vi "参数设置页.vi"() -> ()   [LabVIEW 2016, in "斯坦道CODMn新电路板.lvlib"]
uses:
  <vilib>/Plasmionique/MB Master/MB_Master/MB_Master.lvclass
  <vilib>/ptbypt/NI_PtbyPt.lvlib
panel:
  in  "标样核查自动补测":bool caption="通讯连接"
  in  "跨度核查自动补测":bool caption="通讯连接"
  in  "零点核查自动补测":bool caption="通讯连接"
  in  "标样核查标液偏差":dbl caption="标样核查标液偏差："
  in  "跨度核查标液偏差":dbl caption="跨度核查标液偏差："
  in  "零点核查标液偏差":dbl caption="零点核查标液偏差："
  out "曲线截距 2":dbl caption="曲线截距：" format="%#.6f"
  out "曲线斜率 2":dbl caption="曲线斜率：" format="%#.6f"
  out "二次多项式系数 2":dbl caption="二次多项式系数：" format="%#.6f"
  out "error out":errorcluster
  in  "公式切换阈值滴定数(0~9999)":dbl
  in  "自动测试量程配置":T2={"水样测试量程模式"=enum."H", "标样核查量程模式"=enum."H", "零点核查量程模式"=enum."H", "跨度核查量程模式"=enum."H", "空白测试量程模式"=enum."H", "平行样测试量程模式"=enum."H", "加标回收量程模式"=enum."H", "空白校准量程模式"=enum."H", "标样校准量程模式"=enum."H"}
  out "数据刷新时间":string
  in  "通讯连接":bool
  out "MB table":enum32{"Serial", "TCP"}(tab)
  in  "请选择串口:":refnum<visa-resource-name>
  in  "IP":string="127.0.0.1"
  in  "PORT":string="1001"
  in  "通信方式选择":enum16{"串口", "TCP"}(ring)
  in  "刷新":bool
  in  "测量模式":T3(ring)
  in  "参数下拉列表":u16(ring) items=["CODMn"]
  in  "量程下拉列表":enum16{"低量程", "高量程"}(ring)
  in  "流程路径":path=path "data/流程.xml"
  out "阈值（高->低）":dbl caption="阈值（高->低）："
  out "阈值（低->高）":dbl caption="阈值（低->高）："
  out "量程下限":dbl caption="量程下限："
  out "量程上限":dbl caption="量程上限："
  out "检出限":dbl caption="检出限："
  out "曲线截距":dbl caption="曲线截距：" format="%#.6f"
  out "曲线斜率":dbl caption="曲线斜率：" format="%#.6f"
  out "二次多项式系数":dbl caption="二次多项式系数：" format="%#.6f"
  out "消解时长":dbl caption="消解时长："
  out "消解温度":dbl caption="消解温度："
  out "测量精度":dbl caption="测量精度："
  in  "标样核查标液浓度":dbl caption="标样核查标液浓度："
  in  "跨度核查标液浓度":dbl caption="跨度核查标液浓度："
  in  "零点核查标液浓度":dbl caption="零点核查标液浓度："
  in  "跨度值":dbl caption="跨度值："
  # "日质控自动补测设置"
  # "±"
  # "%"
  # "%"
  # "第一段线性公式"
  # "第二段线性公式"
  # "mg/L"
  # "mg/L"
  # "mg/L"
  # "mg/L"
  # "mg/L"
  # "min"
  # "℃"
  # "mg/L"
  # "mg/L"
  # "mg/L"
  # "mg/L"
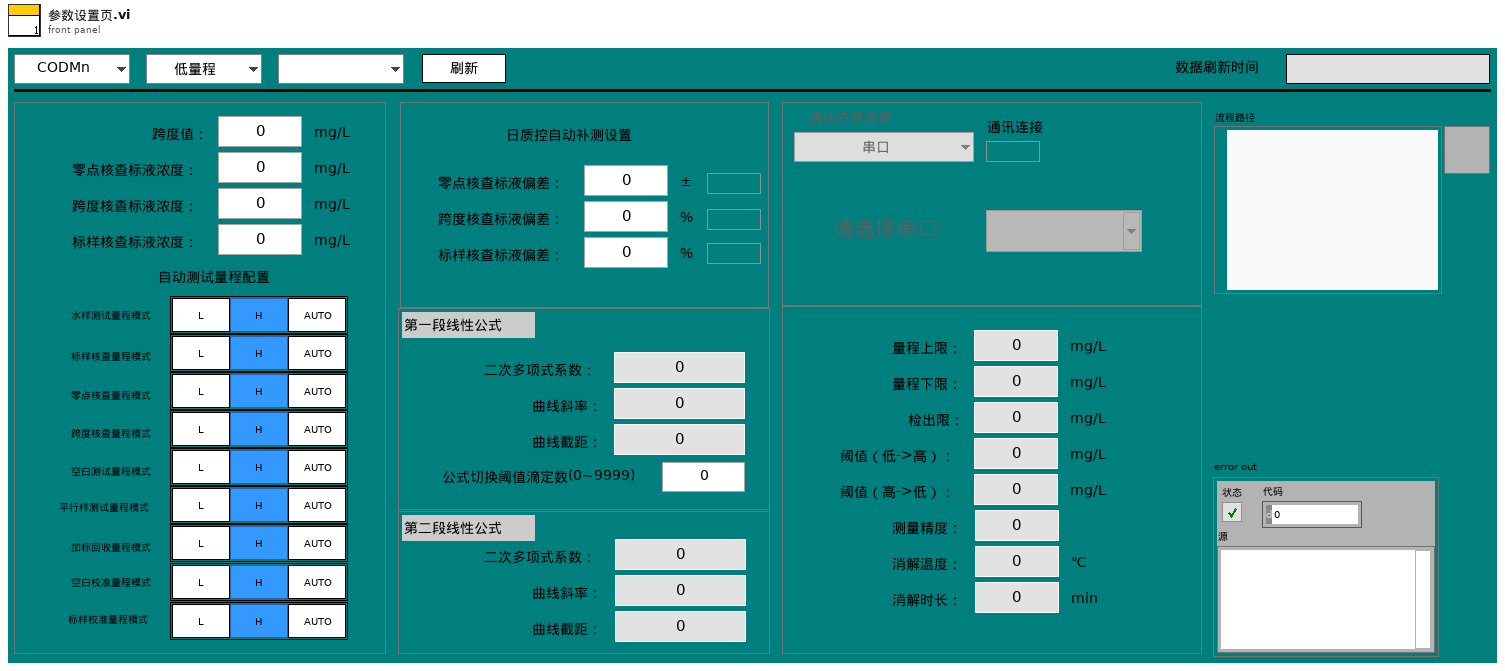
[diagram p1: front panel]
types:
  T1 = typedef "量程选择控件.ctl" = enum32{"L", "H", "AUTO"}
  T2 = cluster{"水样测试量程模式":T1, "标样核查量程模式":T1, "零点核查量程模式":T1, "跨度核查量程模式":T1, "空白测试量程模式":T1, "平行样测试量程模式":T1, "加标回收量程模式":T1, "空白校准量程模式":T1, "标样校准量程模式":T1}
  T3 = enum16{"", "水样测量", "标样核查", "零点核查", "跨度核查", "空白测试", "平行样测试", "加标回收"}
  T4 = enum8{"Enabled", "Disabled", "Disabled and Grayed Out"}
  T5 = cluster{"系统时间":timestamp, "工作状态":u16, "测量模式":enum16{"待机", "连续模式", "周期模式", "定点模式", "受控模式", "手动模式"}, "告警代码":u16, "故障代码":u16, "日志代码":u16, "软件版本":u16, "A":sgl, "B":sgl, "K":sgl, "当前滴定数":sgl, "T":sgl, "H":sgl, "id":u16, "flowid":u16, "量程":u16, "加热实时温度":sgl, "当前ORP值":sgl, "运行时间":sgl, "当前步骤剩余时间":sgl, "结束滴定数":sgl, "注射泵保温温度":sgl, "匹配滴定数X0":u16, "X^2":sgl, "X":sgl, "B 2":sgl, "光值1":sgl, "光值2":sgl, "光值3":sgl, "光值4":sgl, "光值5":sgl, "光值6":sgl, "光值7":sgl, "光值8":sgl}
  T6 = cluster{"检出限":dbl, "测量精度":dbl, "上限":dbl, "下限":dbl, "阈值（低->高）":dbl, "阈值（高->低）":dbl}
  T7 = cluster{"标液浓度1":dbl, "测量吸光度1":dbl, "样品1启用":bool, "标液浓度2":dbl, "测量吸光度2":dbl, "样品2启用":bool, "标液浓度3":dbl, "测量吸光度3":dbl, "样品3启用":bool, "标液浓度4":dbl, "测量吸光度4":dbl, "样品4启用":bool, "标液浓度5":dbl, "测量吸光度5":dbl, "样品5启用":bool, "模型":enum32{"线性", "多项式", "折线"}, "精度":dbl, "XY图":cluster{"X Values":dbl[], "Y Values":dbl[]}[], "拟合公式":string, "r^2":dbl, "标样一校准时间":timestamp, "标样二校准时间":timestamp, "标样三校准时间":timestamp, "标样四校准时间":timestamp, "标样五校准时间":timestamp, "二次方程":cluster{"c":dbl, "x":dbl, "x^2":dbl}, "标定时间":timestamp, "拟合公式 2":string, "r^2 2":dbl}[][]
  T8 = cluster{"运行模式":enum16{"维护模式", "常规模式", "应急模式", "质控模式"}, "质控频次":enum16{"关闭", "每天", "星期一", "星期二", "星期三", "星期四", "星期五", "星期六", "星期日"}, "空白核查时间":u16, "跨度核查时间":u16, "测量间隔":u16}
  T9 = cluster{"标液浓度1":dbl, "测量吸光度1":dbl, "样品1启用":bool, "标液浓度2":dbl, "测量吸光度2":dbl, "样品2启用":bool, "标液浓度3":dbl, "测量吸光度3":dbl, "样品3启用":bool, "标液浓度4":dbl, "测量吸光度4":dbl, "样品4启用":bool, "标液浓度5":dbl, "测量吸光度5":dbl, "样品5启用":bool, "模型":enum32{"线性", "多项式", "折线"}, "精度":dbl, "XY图":cluster{"X Values":dbl[], "Y Values":dbl[]}[], "拟合公式":string, "r^2":dbl, "标样一校准时间":timestamp, "标样二校准时间":timestamp, "标样三校准时间":timestamp, "标样四校准时间":timestamp, "标样五校准时间":timestamp, "二次方程":cluster{"c":dbl, "x":dbl, "x^2":dbl}, "标定时间":timestamp, "拟合公式 2":string, "r^2 2":dbl}
  T10 = cluster{"测量量程":sgl, "测量检出限":sgl, "测量精度":sgl, "测量间隔":sgl, "消解温度":sgl, "消解时长":sgl, "三项式系数":sgl, "二次多项式系数":sgl, "曲线斜率":sgl, "曲线截距":sgl, "线性相关系数":sgl, "空白校准时间":timestamp, "标样校准时间":timestamp, "测量信号值":sgl, "稀释倍数":sgl, "量程系数":sgl}
  T11 = cluster{"偏心轮校准参数":dbl, "运行速度(修改需要重启)":u16, "加热温度(校准参数) ":dbl, "告警温度":dbl, "加热超时时间:(单位/秒)":dbl, "K p":dbl, "K i":dbl, "K d":dbl, "ILimitUp":dbl, "ILimitDown":dbl}
  T12 = cluster{"泵类型":u8, "阀数量":u8, "纯水通道":u8, "废液通道":u8, "进样速度":u16, "出样速度":u16, "滴定速度":u16, "注射泵保温温度L":u8, "注射泵保温温度H":u8, "注射泵加热超时时间":u16, "是否存在液位检测板":u16, "A值告警下限值":u16, "A值告警上限值":u16, "B值告警下限值":u16, "B值告警上限值":u16, "AB跨度告警值":u16, "阀配置:":u8, "滴定等待时间":u16, "滴定吸光度斜率":dbl}
  T13 = cluster{"跨度值":dbl, "零点标准液浓度":dbl, "跨度标准液浓度":dbl, "标准液标准浓度":dbl, "零点标准液偏差":dbl, "跨度标准液偏差":dbl, "标准液标准偏差":dbl}
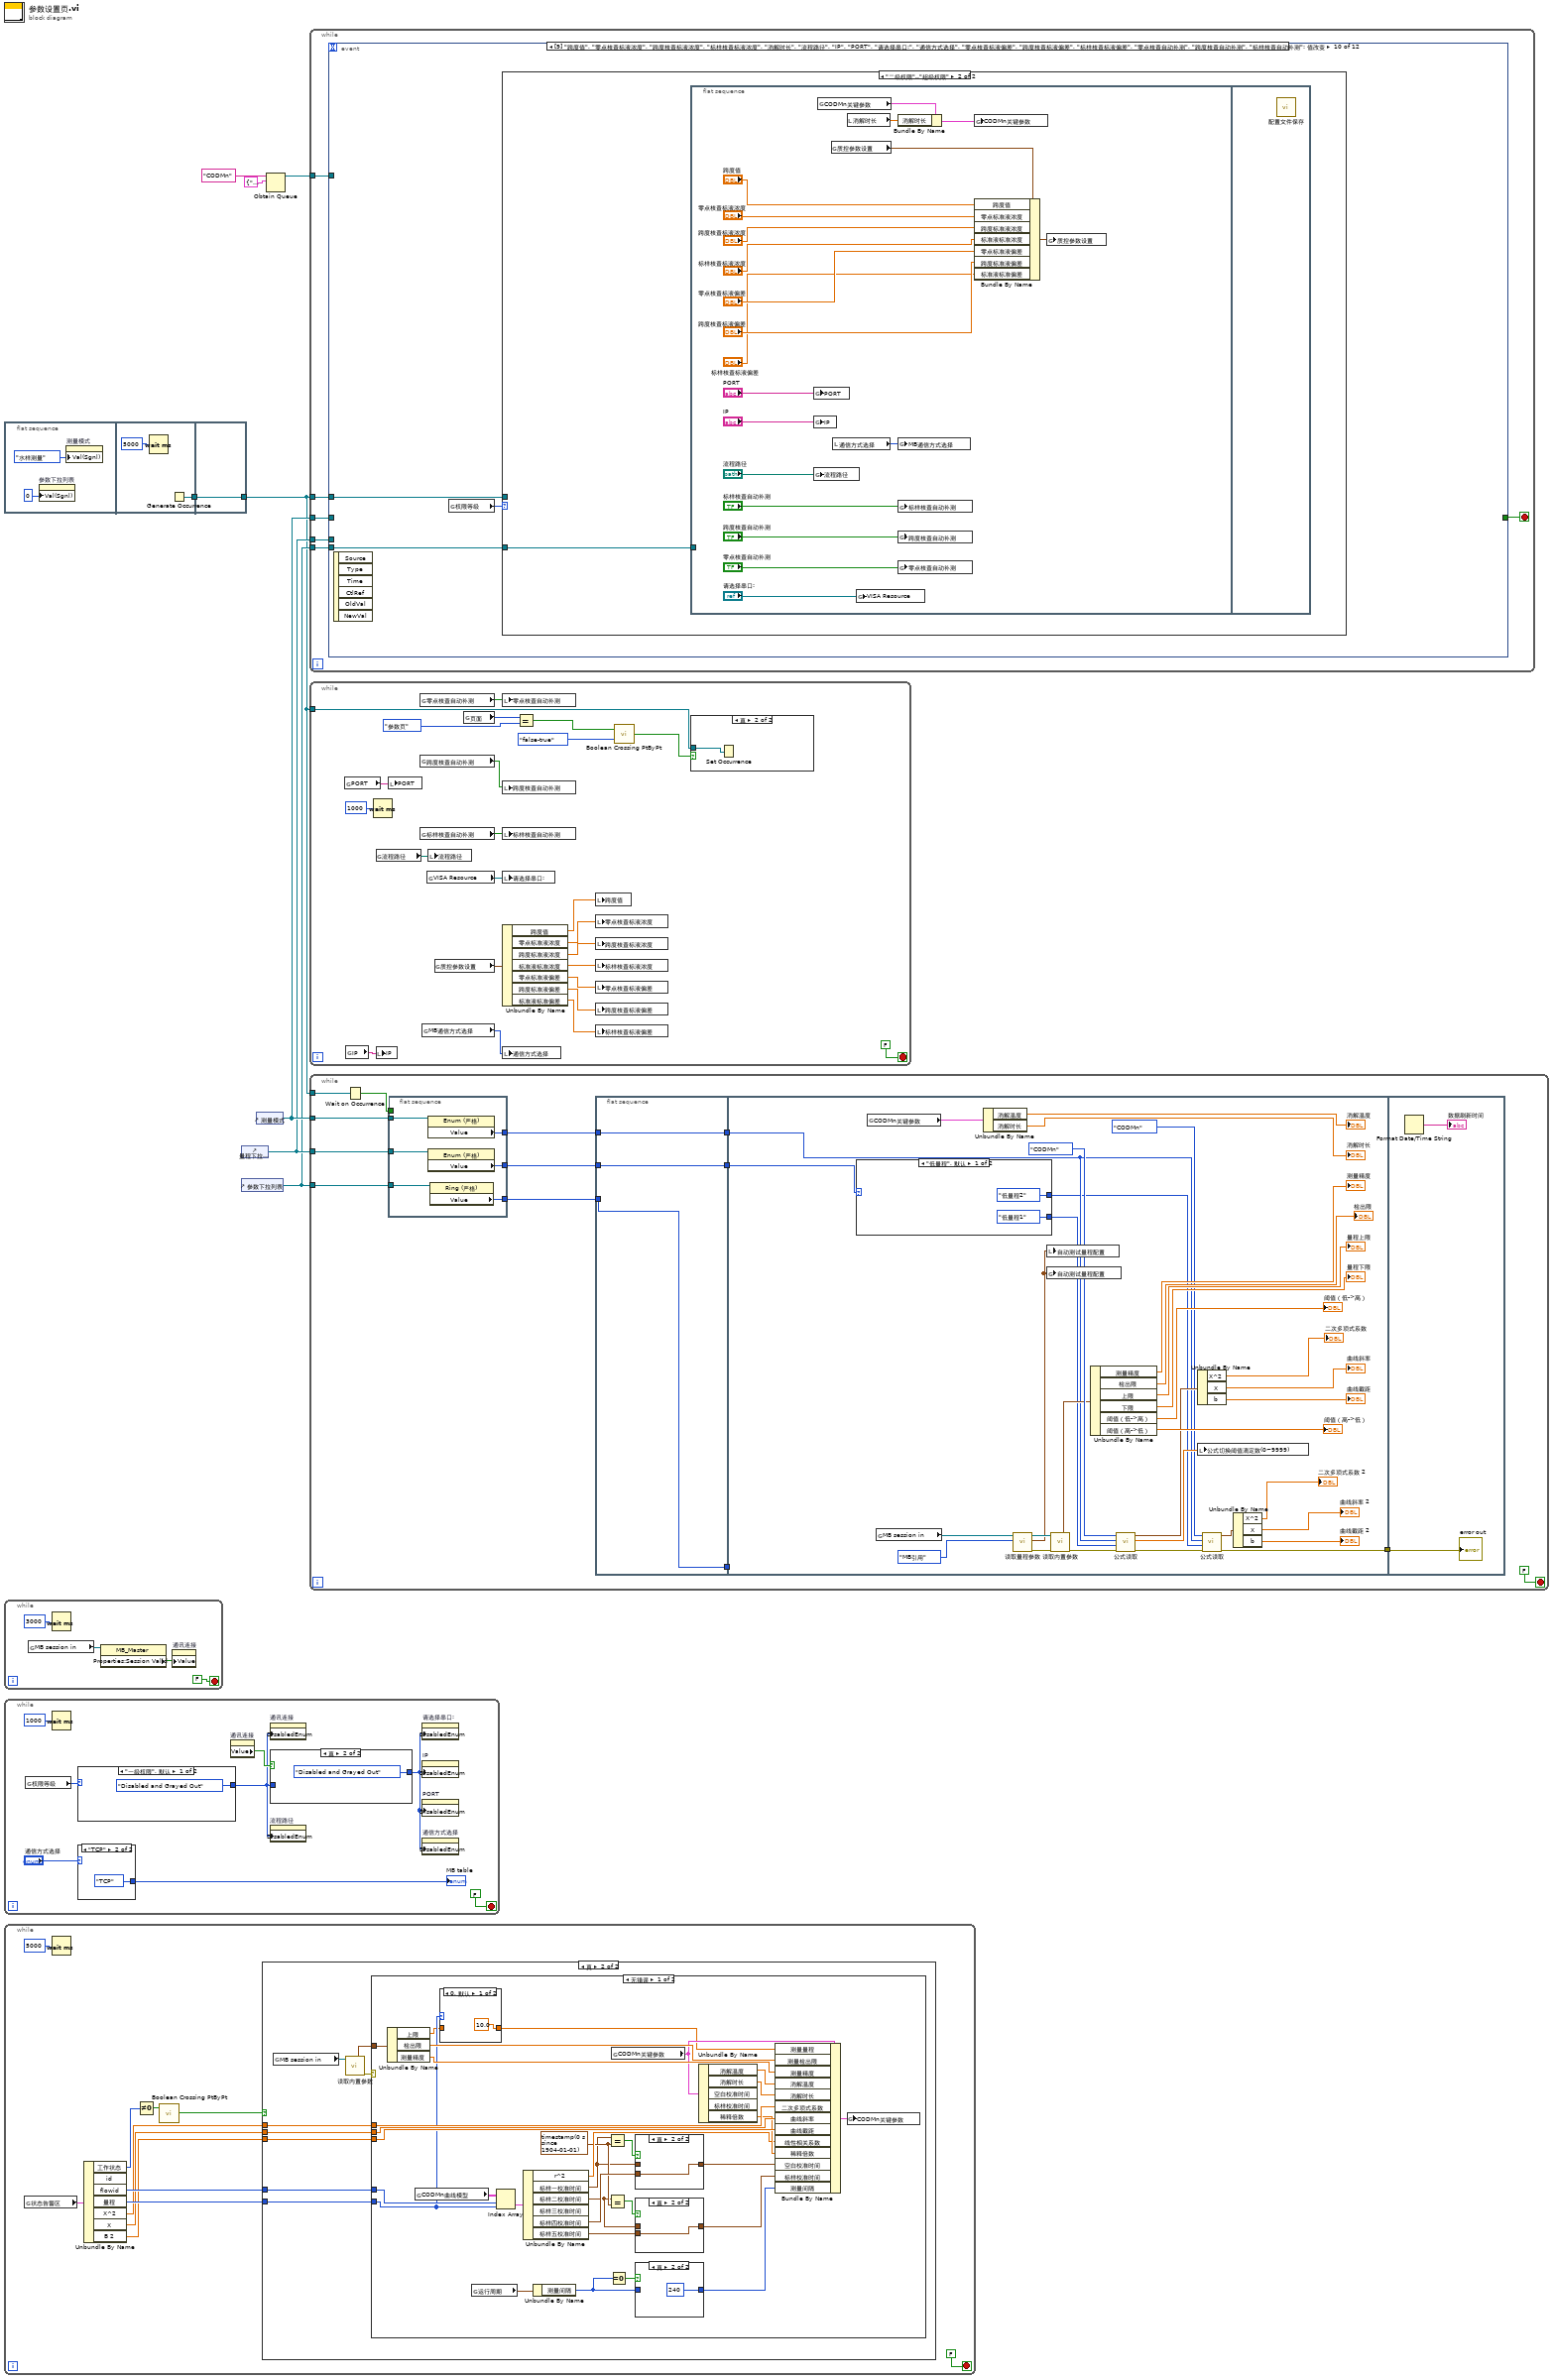
[diagram p0: block diagram]
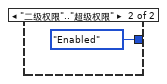
[diagram p9: hidden frame]
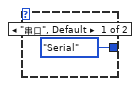
[diagram p10: hidden frame]
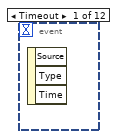
[diagram p12: hidden frame]
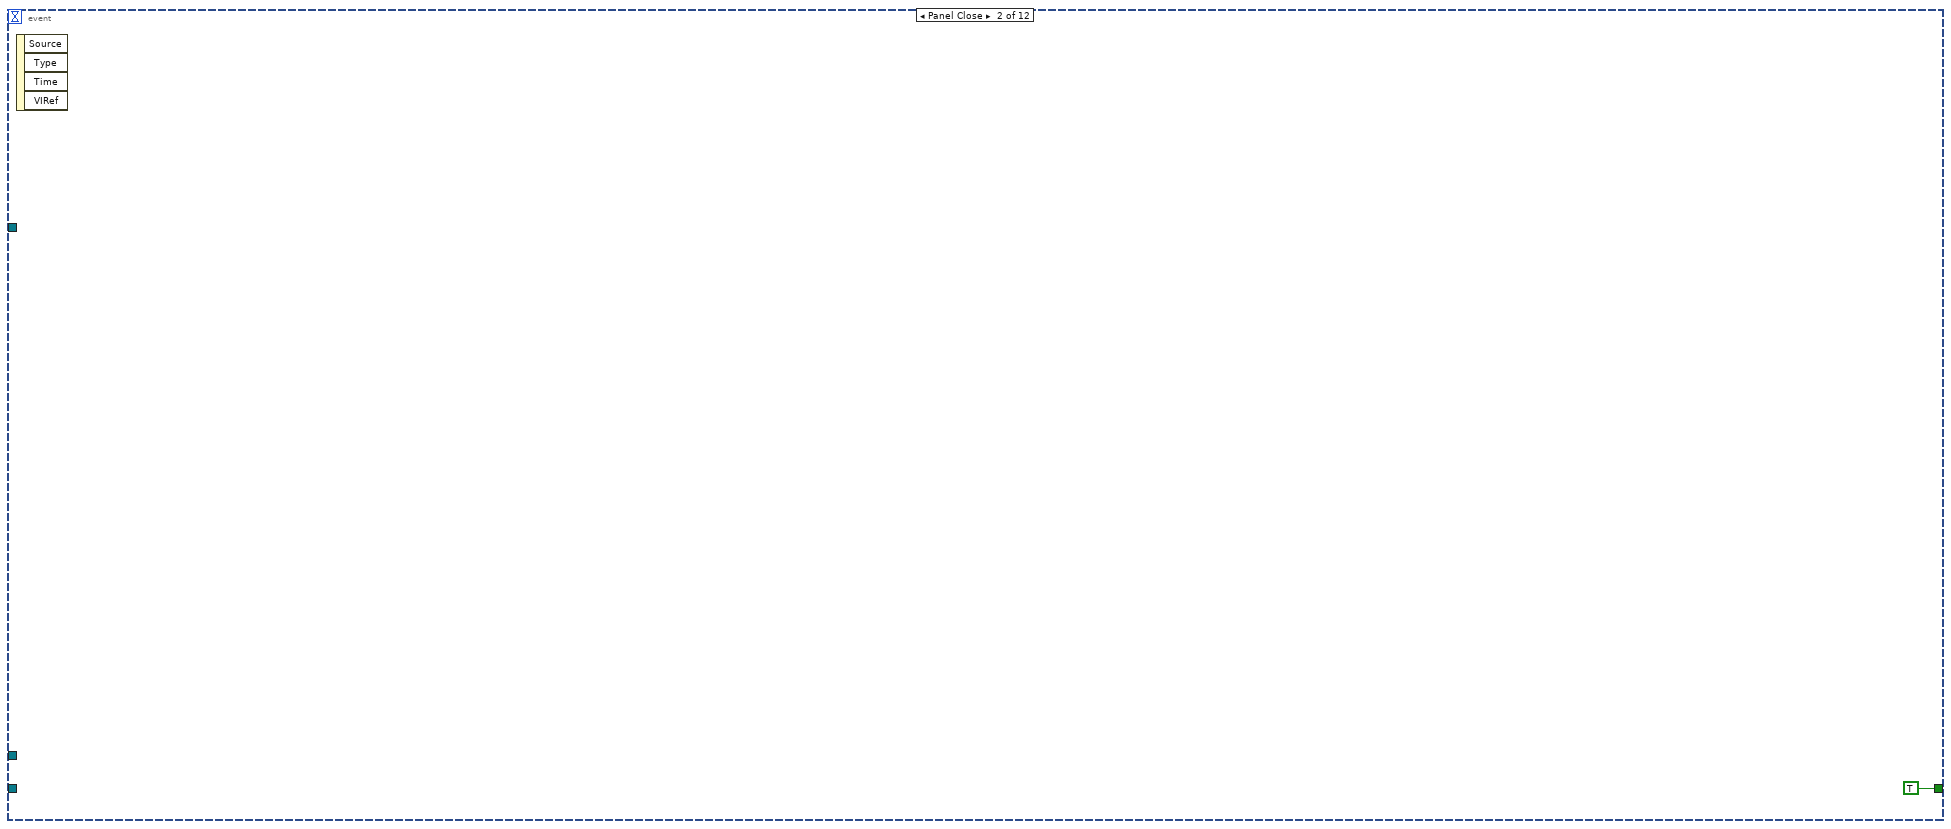
[diagram p13: hidden frame]
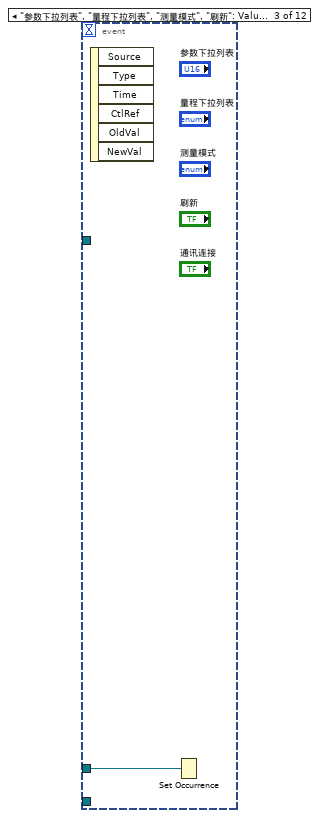
[diagram p14: hidden frame]
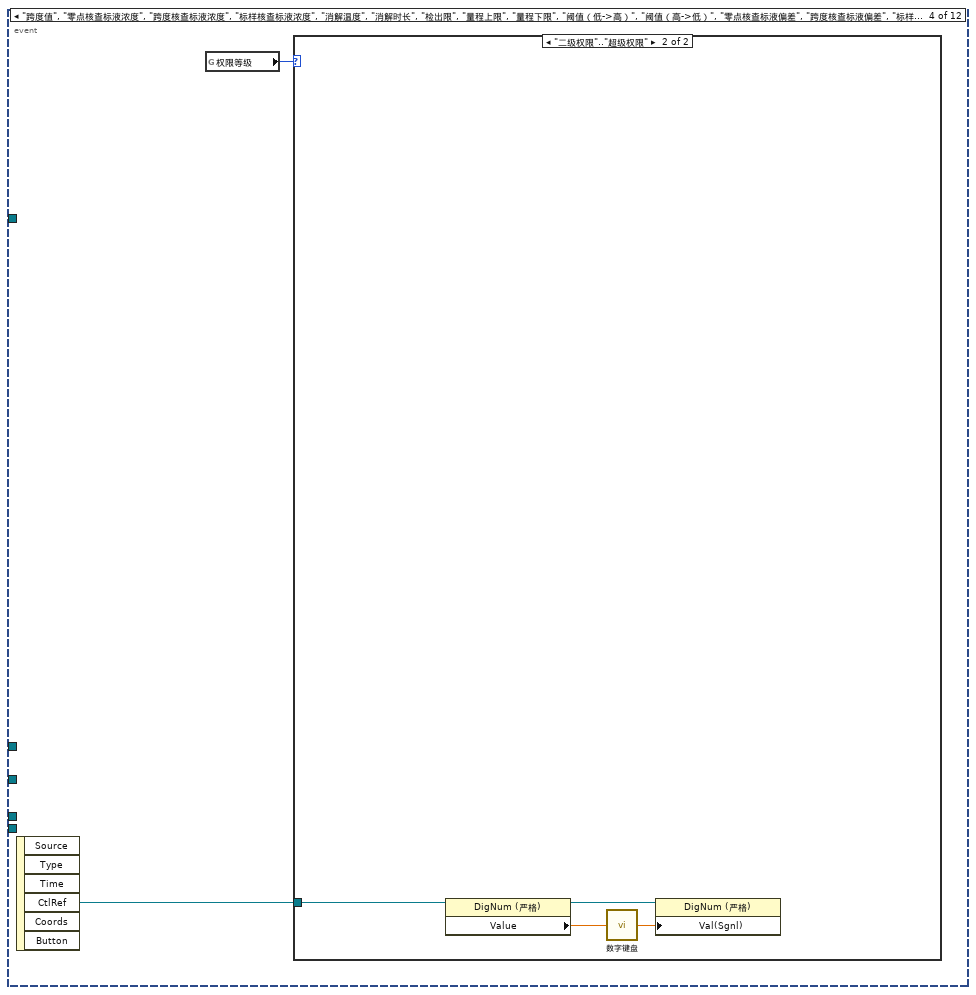
[diagram p15: hidden frame]
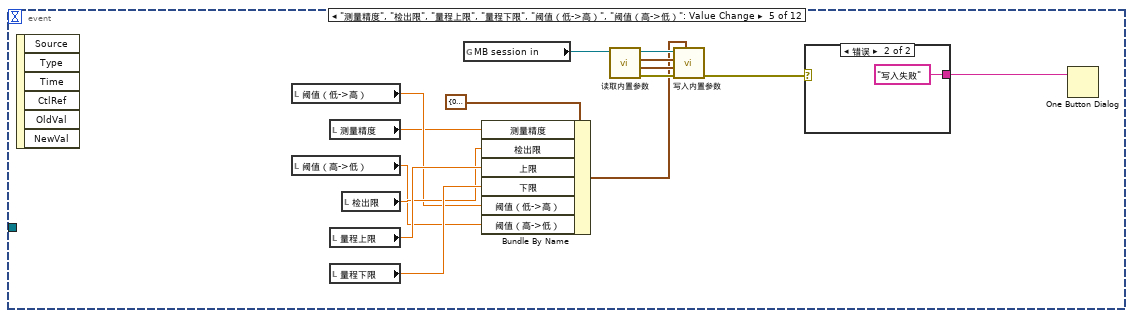
[diagram p17: hidden frame]
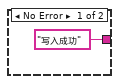
[diagram p18: hidden frame]
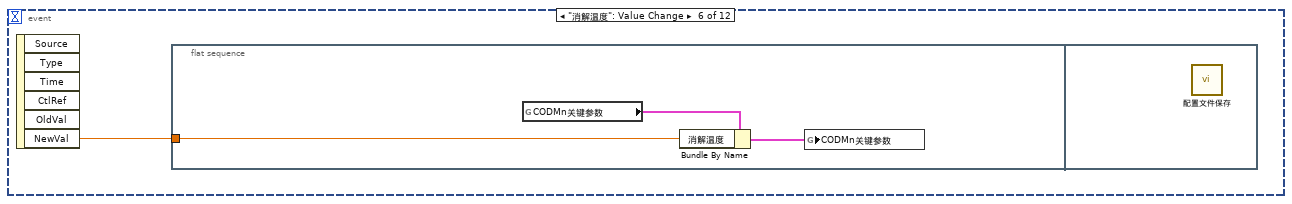
[diagram p19: hidden frame]
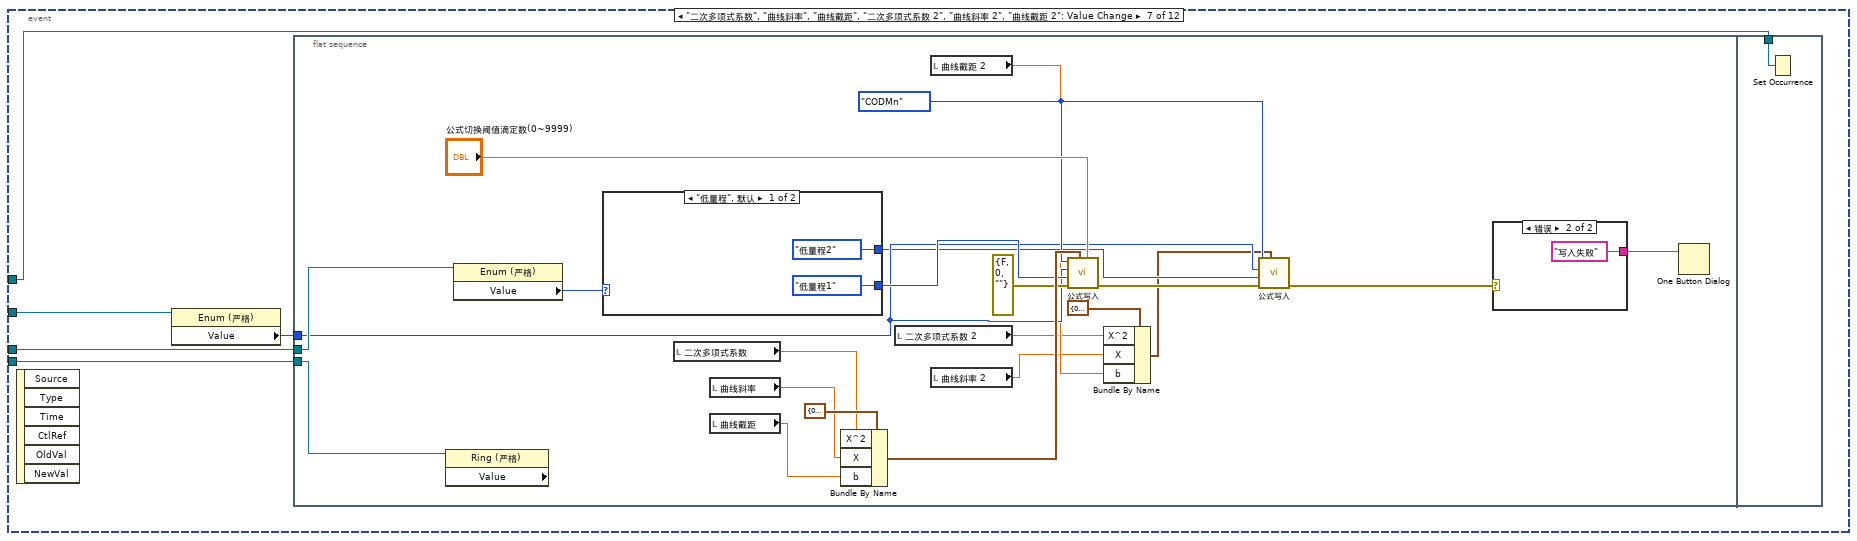
[diagram p20: hidden frame]
diagram:
  n1 = flat-sequence {
    tunnel: [w12] -> w8
    tunnel: [w13] -> w1
    tunnel: w8 -> [w13]
    frame #0 {
      n2 = property on="参数下拉列表" class="Ring (严格)"("Val(Sgnl)"=u16 0 ("值(信号)")) -> ()  [unwired: 2 in, 2 out]
      n3 = property on="测量模式" class="Enum (严格)"("Val(Sgnl)"=T3."水样测量" ("值(信号)")) -> ()  [unwired: 2 in, 2 out]
    }
    frame #1 {
      n4 = Wait (ms)(milliseconds to wait=u32 5000 ("等待时间（毫秒）")) -> ()  [unwired: 1 out]
      n5 = Generate Occurrence() -> (w12:refnum<k4>)
    }
    frame #2 {
    }
  }
  n6 = while {
    stop <- FALSE stop-if-true
    n7 = global read "VARCODMn全局变量.vi" "MB session in"() -> (w16:refnum<class "MB_Master.lvclass">)
    n8 = Wait (ms)(milliseconds to wait=u32 3000 ("等待时间（毫秒）")) -> ()  [unwired: 1 out]
    n9 = property class="MB_Master"(reference=w16) -> ("Properties:Session Valid"=w15:bool)  [unwired: 1 in, 2 out]
    n10 = property on="通讯连接" class="Bool (严格)"("Value"=w15) -> ()  [unwired: 2 in, 2 out]
  }
  n11 = while {
    stop <- FALSE stop-if-true
    n12 = global read "VARCODMn全局变量.vi" "权限等级"() -> (w18:enum16{"一级权限", "二级权限", "三级权限", "超级权限"})
    n13 = Wait (ms)(milliseconds to wait=u32 1000 ("等待时间（毫秒）")) -> ()  [unwired: 1 out]
    n14 = case shown="\"一级权限\", 默认" w18 {
      tunnel: [T4."Disabled and Grayed Out" ("禁用") T4."Enabled" ("禁用")] -> w19
      frame "一级权限", Default {
      }
      frame "二级权限".."超级权限" {
      }
    }
    n15 = case shown="\"TCP\"" "通信方式选择" {
      tunnel: [enum32{"Serial", "TCP"}."Serial" ("MB table") enum32{"Serial", "TCP"}."TCP" ("MB table")] -> w21
      frame "串口", Default {
      }
      frame "TCP" {
      }
    }
    "MB table" <- w21
    n16 = property on="通讯连接" class="Bool (严格)"() -> ("Value"=w23:bool)  [unwired: 2 in, 2 out]
    n17 = property on="通讯连接" class="Bool (严格)"("DisabledEnum"=w19) -> ()  [unwired: 2 in, 2 out]
    n18 = case shown="真" w23 {
      tunnel: [w30 T4."Disabled and Grayed Out" ("禁用")] -> w22
      tunnel: w19 -> [w30 _]
      frame False {
      }
      frame True {
      }
    }
    n19 = property on="流程路径" class="Path"("DisabledEnum"=w19) -> ()  [unwired: 2 in, 2 out]
    n20 = property on="请选择串口:" class="VISAName"("DisabledEnum"=w22) -> ()  [unwired: 2 in, 2 out]
    n21 = property on="IP" class="Str"("DisabledEnum"=w22) -> ()  [unwired: 2 in, 2 out]
    n22 = property on="PORT" class="Str"("DisabledEnum"=w22) -> ()  [unwired: 2 in, 2 out]
    n23 = property on="通信方式选择" class="Enum (严格)"("DisabledEnum"=w22) -> ()  [unwired: 2 in, 2 out]
  }
  n24 = while {
    stop <- FALSE stop-if-true
    n25 = global read "VARCODMn全局变量.vi" "状态告警区"() -> (w42:T5)
    n26 = Wait (ms)(milliseconds to wait=u32 5000 ("等待时间（毫秒）")) -> ()  [unwired: 1 out]
    n27 = Unbundle By Name(w42) -> ("工作状态"=w41:u16, "flowid"=w35:u16, "量程"=w36:u16, "X^2"=w34:sgl, "X"=w33:sgl, "B 2"=w32:sgl)  [unwired: 1 out]
    n28 = Not Equal To 0?(x=w41) -> (x != 0?=w40:bool)
    n29 = call <vilib>:"Boolean Crossing PtByPt.vi"("input"=w40) -> ("crossing"=w39:bool)  [unwired: 2 in]
    n30 = case shown="真" w39 {
      tunnel: w36 -> [_ w48]
      tunnel: w35 -> [_ w47]
      tunnel: w34 -> [_ w46]
      tunnel: w33 -> [_ w45]
      tunnel: w32 -> [_ w44]
      frame False {
      }
      frame True {
        n31 = global read "VARCODMn全局变量.vi" "MB session in"() -> (w50:refnum<class "MB_Master.lvclass">)
        n32 = call "读取内置参数.vi"("MB session in"=w50) -> ("error out"=w43:errorcluster, "量程参数读取"=w49:T6)  [unwired: 6 in, 3 out]
        n33 = case shown="无错误" w43 {
          tunnel: w49 -> [w81 _]
          tunnel: w46 -> [w80 _]
          tunnel: w45 -> [w79 _]
          tunnel: w44 -> [w78 _]
          tunnel: w48 -> [w53 _]
          tunnel: w47 -> [w71 _]
          frame No Error {
            w60 = timestamp(0 s since 1904-01-01) ("y")
            n34 = Unbundle By Name(w81) -> ("上限"=w52:dbl, "检出限"=w77:dbl, "测量精度"=w76:dbl)
            n35 = global read "校准数据全局变量.vi" "CODMn曲线模型"() -> (w72:T7)
            n36 = case shown="0, 默认" w53 {
              tunnel: w52 -> [_ w83]
              tunnel: [10.0 ("上限") w83] -> w51
              frame 0, Default {
              }
              frame 1 {
              }
            }
            n37 = global read "CODMn断电保存全局变量.vi" "运行周期"() -> (w67:T8)
            n38 = Index Array(array=w72, index (row)=w71, index (col)=w53) -> (element=w70:T9)
            n39 = Unbundle By Name(w70) -> ("r^2"=w68:dbl, "标样一校准时间"=w56:timestamp, "标样二校准时间"=w57:timestamp, "标样四校准时间"=w61:timestamp, "标样五校准时间"=w58:timestamp)  [unwired: 1 out]
            n40 = Unbundle By Name(w67) -> ("测量间隔"=w63:u16)
            n41 = Equal?(x=w56, y=w60) -> (x = y?=w62:bool)
            n42 = Equal?(x=w57, y=w60) -> (x = y?=w59:bool)
            n43 = Equal To 0?(x=w63) -> (x = 0?=w65:bool)
            n44 = global read "CODMn断电保存全局变量.vi" "CODMn关键参数"() -> (w66:T10)
            n45 = case shown="真" w62 {
              tunnel: w61 -> [_ w87]
              tunnel: [w86 w87] -> w55
              tunnel: w56 -> [w86 _]
              frame False {
              }
              frame True {
              }
            }
            n46 = case shown="真" w59 {
              tunnel: w58 -> [_ w85]
              tunnel: [w84 w85] -> w54
              tunnel: w57 -> [w84 _]
              frame False {
              }
              frame True {
              }
            }
            n47 = case shown="真" w65 {
              tunnel: [w88 u16 240 ("测量间隔")] -> w64
              tunnel: w63 -> [w88 _]
              frame False {
              }
              frame True {
              }
            }
            n48 = Unbundle By Name(w66) -> ("消解温度"=w75:sgl, "消解时长"=w74:sgl, "稀释倍数"=w69:sgl)  [unwired: 2 out]
            n49 = Bundle By Name(cluster=w66, "测量量程"=w51, "测量检出限"=w77, "测量精度"=w76, "消解温度"=w75, "消解时长"=w74, "二次多项式系数"=w80, "曲线斜率"=w79, "曲线截距"=w78, "线性相关系数"=w68, "稀释倍数"=w69, "空白校准时间"=w55, "标样校准时间"=w54, "测量间隔"=w64) -> (w73:T10)
            n50 = global write "CODMn断电保存全局变量.vi" "CODMn关键参数"(w73) -> ()
          }
          frame Error {
          }
        }
      }
    }
  }
  n51 = control-ref of="量程下拉列表"() -> (w4:refnum<vi>)
  n52 = control-ref of="参数下拉列表"() -> (w3:refnum<vi>)
  n53 = control-ref of="测量模式"() -> (w5:refnum<vi>)
  n54 = Obtain Queue(name (unnamed)="CODMn" ("名称（未命名）"), element data type=cluster{"命令":string, "data":variant} {"命令"="", "data"=variant}) -> (queue out=w6:refnum<queue>)  [unwired: 3 in, 2 out]
  n55 = while {
    tunnel: w1 -> [w94]
    tunnel: w3 -> [w93]
    tunnel: w6 -> [w92]
    tunnel: w5 -> [w91]
    tunnel: w4 -> [w90]
    stop <- w95 stop-if-true
    n56 = event shown="[9] \"跨度值\", \"零点核查标液浓度\", \"跨度核查标液浓度\", \"标样核查标液浓度\", \"消解时长\", \"流程路径\", \"IP\", \"PORT\", \"请选择串口:\", \"通信方式选择\", \"零点核查标液偏差\", \"跨度核查标液偏差\", \"标样核查标液偏差\", \"零点核查自动补测\", \"跨度核查自动补测\", \"标样核查自动补测\": 值改变" {
      selector: _ -> [_ _ _ _ _ _ _ _ _ _ _ _]
      dyn-events: _ -> [_ _ _ _ _ _ _ _ _ _ _ _]
      timeout: _ -> [_ _ _ _ _ _ _ _ _ _ _ _]
      tunnel: [_ TRUE _ _ _ _ _ _ _ _ _ _] -> w95
      tunnel: w94 -> [_ _ w97 _ _ _ w125 _ _ w172 w197 _]
      tunnel: w93 -> [_ _ _ _ _ _ w129 _ _ w174 _ _]
      tunnel: w92 -> [_ _ _ _ _ _ _ _ _ _ _ w203]
      tunnel: w91 -> [_ _ _ _ _ _ w128 _ _ _ _ _]
      tunnel: w90 -> [_ _ _ _ _ _ w126 _ _ _ _ _]
      event Timeout {
        n57 = event-data() -> ()  [unwired: 1 in, 3 out]
      }
      event Panel Close {
        n58 = event-data() -> ()  [unwired: 1 in, 4 out]
      }
      event "参数下拉列表", "量程下拉列表", "测量模式", "刷新": Value Change {
        n59 = event-data() -> ()  [unwired: 1 in, 6 out]
        n60 = Set Occurrence(w97) -> ()
      }
      event "跨度值", "零点核查标液浓度", "跨度核查标液浓度", "标样核查标液浓度", "消解温度", "消解时长", "检出限", "量程上限", "量程下限", "阈值（低->高）", "阈值（高->低）", "零点核查标液偏差", "跨度核查标液偏差", "标样核查标液偏差": Mouse Down {
        n61 = event-data() -> ("CtlRef"=w99:refnum<vi>)  [unwired: 1 in, 5 out]
        n62 = global read "VARCODMn全局变量.vi" "权限等级"() -> (w98:enum16{"一级权限", "二级权限", "三级权限", "超级权限"})
        n63 = case shown="\"二级权限\"..\"超级权限\"" w98 {
          tunnel: w99 -> [_ w103]
          frame "一级权限", Default {
          }
          frame "二级权限".."超级权限" {
            n64 = property class="DigNum (严格)"(reference=w103) -> (reference out=w101:refnum<vi>, "Value"=w102:dbl)  [unwired: 1 in, 1 out]
            n65 = call "数字键盘.vi"("OldNumber"=w102) -> ("NewNumber"=w100:dbl)
            n66 = property class="DigNum (严格)"(reference=w101, "Val(Sgnl)"=w100) -> ()  [unwired: 1 in, 2 out]
          }
        }
      }
      event "测量精度", "检出限", "量程上限", "量程下限", "阈值（低->高）", "阈值（高->低）": Value Change {
        n67 = event-data() -> ()  [unwired: 1 in, 6 out]
        n68 = local read "阈值（低->高）"() -> (w115:dbl)
        n69 = local read "阈值（高->低）"() -> (w114:dbl)
        n70 = local read "测量精度"() -> (w113:dbl)
        n71 = local read "量程上限"() -> (w118:dbl)
        n72 = local read "量程下限"() -> (w117:dbl)
        n73 = local read "检出限"() -> (w116:dbl)
        n74 = global read "VARCODMn全局变量.vi" "MB session in"() -> (w111:refnum<class "MB_Master.lvclass">)
        n75 = Bundle By Name(cluster=T6 {"检出限"=0.0, "测量精度"=0.0, "上限"=0.0, "下限"=0.0, "阈值（低->高）"=0.0, "阈值（高->低）"=0.0} ("量程参数读取"), "测量精度"=w113, "检出限"=w116, "上限"=w118, "下限"=w117, "阈值（低->高）"=w115, "阈值（高->低）"=w114) -> (w104:T6)
        n76 = call "读取内置参数.vi"("MB session in"=w111) -> ("error out"=w107:errorcluster, "float"=w108:T11, "外设配置"=w109:T12, "MB session out"=w110:refnum<class "MB_Master.lvclass">)  [unwired: 6 in, 1 out]
        n77 = call "写入内置参数.vi"("量程参数读取"=w104, "error in (no error)"=w107, "float"=w108, "外设配置"=w109, "MB session in"=w110) -> ("error out"=w106:errorcluster)  [unwired: 5 in, 1 out]
        n78 = case shown="错误" w106 {
          tunnel: ["写入成功" "写入失败"] -> w112
          frame No Error {
          }
          frame Error {
          }
        }
        n79 = One Button Dialog(message=w112) -> ()  [unwired: 1 in, 1 out]
      }
      event "消解温度": Value Change {
        n80 = event-data() -> ("NewVal"=w121:dbl)  [unwired: 1 in, 5 out]
        n81 = flat-sequence {
          tunnel: w121 -> [w124]
          frame #0 {
            n82 = global read "CODMn断电保存全局变量.vi" "CODMn关键参数"() -> (w122:T10)
            n83 = Bundle By Name(cluster=w122, "消解温度"=w124) -> (w123:T10)
            n84 = global write "CODMn断电保存全局变量.vi" "CODMn关键参数"(w123) -> ()
          }
          frame #1 {
            n85 = call "配置文件保存.vi"() -> ()  [unwired: 12 in]
          }
        }
      }
      event "二次多项式系数", "曲线斜率", "曲线截距", "二次多项式系数 2", "曲线斜率 2", "曲线截距 2": Value Change {
        n86 = event-data() -> ()  [unwired: 1 in, 6 out]
        n87 = property class="Enum (严格)"(reference=w128) -> ("Value"=w127:T3)  [unwired: 1 in, 2 out]
        n88 = flat-sequence {
          tunnel: w129 -> [w151]
          tunnel: w127 -> [w137]
          tunnel: w126 -> [w150]
          tunnel: w125 -> [w158]
          frame #0 {
            w138 = enum16{"CODMn"}."CODMn" ("测量参数")
            n89 = property class="Ring (严格)" props=["Value"](reference=w151) -> ()  [unwired: 1 in, 3 out]
            n90 = property class="Enum (严格)"(reference=w150) -> ("Value"=w141:enum16{"低量程", "高量程"})  [unwired: 1 in, 2 out]
            n91 = case shown="\"低量程\", 默认" w141 {
              tunnel: [enum16{"低量程1", "低量程2", "高量程1", "高量程2"}."低量程1" ("量程") enum16{"低量程1", "低量程2", "高量程1", "高量程2"}."高量程1" ("量程")] -> w140
              tunnel: [enum16{"低量程1", "低量程2", "高量程1", "高量程2"}."低量程2" ("量程") enum16{"低量程1", "低量程2", "高量程1", "高量程2"}."高量程2" ("量程")] -> w136
              frame "低量程", Default {
              }
              frame "高量程" {
              }
            }
            n92 = local read "二次多项式系数"() -> (w147:dbl)
            n93 = local read "曲线斜率"() -> (w146:dbl)
            n94 = local read "曲线截距"() -> (w145:dbl)
            n95 = Bundle By Name(cluster=cluster{"X^2":dbl, "X":dbl, "b":dbl} {"X^2"=0.0, "X"=0.0, "b"=0.0} ("公式"), "X^2"=w147, "X"=w146, "b"=w145) -> (w148:cluster{"X^2":dbl, "X":dbl, "b":dbl})
            n96 = local read "二次多项式系数 2"() -> (w133:dbl)
            n97 = local read "曲线截距 2"() -> (w135:dbl)
            n98 = local read "曲线斜率 2"() -> (w134:dbl)
            n99 = call "公式写入.vi"("临界滴定数"="公式切换阈值滴定数(0~9999)", "公式"=w148, "error in (no error)"=errorcluster {"status"=FALSE, "code"=0, "source"=""} ("error out"), "量程"=w140, "测量模式"=w137, "测量参数"=w138) -> ("error out"=w139:errorcluster)  [unwired: 5 in]
            n100 = Bundle By Name(cluster=cluster{"X^2":dbl, "X":dbl, "b":dbl} {"X^2"=0.0, "X"=0.0, "b"=0.0} ("公式"), "X^2"=w133, "X"=w134, "b"=w135) -> (w131:cluster{"X^2":dbl, "X":dbl, "b":dbl})
            n101 = call "公式写入.vi"("公式"=w131, "error in (no error)"=w139, "量程"=w136, "测量模式"=w137, "测量参数"=w138) -> ("error out"=w130:errorcluster)  [unwired: 6 in]
            n102 = case shown="错误" w130 {
              tunnel: ["写入成功" "写入失败"] -> w144
              frame No Error {
              }
              frame Error {
              }
            }
            n103 = One Button Dialog(message=w144) -> ()  [unwired: 1 in, 1 out]
          }
          frame #1 {
            n104 = Set Occurrence(w158) -> ()
          }
        }
      }
      event "测量精度": Mouse Down {
        n105 = event-data() -> ("CtlRef"=w160:refnum<vi>)  [unwired: 1 in, 7 out]
        n106 = global read "VARCODMn全局变量.vi" "权限等级"() -> (w159:enum16{"一级权限", "二级权限", "三级权限", "超级权限"})
        n107 = case shown="\"二级权限\"..\"超级权限\"" w159 {
          tunnel: w160 -> [_ w164]
          frame "一级权限", Default {
          }
          frame "二级权限".."超级权限" {
            n108 = property class="DigNum (严格)"(reference=w164) -> (reference out=w162:refnum<vi>, "Value"=w163:dbl)  [unwired: 1 in, 1 out]
            n109 = call "数字键盘.vi"("OldNumber"=w163) -> ("NewNumber"=w161:dbl)
            n110 = property class="DigNum (严格)"(reference=w162, "Val(Sgnl)"=w161) -> ()  [unwired: 1 in, 2 out]
          }
        }
      }
      event "二次多项式系数", "曲线斜率", "曲线截距", "二次多项式系数 2", "曲线斜率 2", "曲线截距 2": Mouse Down {
        n111 = event-data() -> ("CtlRef"=w165:refnum<vi>)  [unwired: 1 in, 7 out]
        n112 = disable-structure shown="启用" {
          disable-tunnel: w165 -> [w167 _]
          frame Disabled {
            n113 = global read "VARCODMn全局变量.vi" "权限等级"() -> (w166:enum16{"一级权限", "二级权限", "三级权限", "超级权限"})
            n114 = case shown="\"三级权限\", \"超级权限\"" w166 {
              tunnel: w167 -> [_ w171]
              frame "一级权限", Default {
              }
              frame "三级权限", "超级权限" {
                n115 = property class="DigNum (严格)"(reference=w171) -> (reference out=w169:refnum<vi>, "Value"=w170:dbl)  [unwired: 1 in, 1 out]
                n116 = call "数字键盘.vi"("OldNumber"=w170) -> ("NewNumber"=w168:dbl)
                n117 = property class="DigNum (严格)"(reference=w169, "Val(Sgnl)"=w168) -> ()  [unwired: 1 in, 2 out]
              }
            }
          }
          frame Enabled {
          }
        }
      }
      event "跨度值", "零点核查标液浓度", "跨度核查标液浓度", "标样核查标液浓度", "消解时长", "流程路径", "IP", "PORT", "请选择串口:", "通信方式选择", "零点核查标液偏差", "跨度核查标液偏差", "标样核查标液偏差", "零点核查自动补测", "跨度核查自动补测", "标样核查自动补测": Value Change {
        n118 = event-data() -> ()  [unwired: 1 in, 6 out]
        n119 = global read "VARCODMn全局变量.vi" "权限等级"() -> (w173:enum16{"一级权限", "二级权限", "三级权限", "超级权限"})
        n120 = case shown="\"二级权限\"..\"超级权限\"" w173 {
          tunnel: w174 -> [_ w176]
          tunnel: w172 -> [w175 _]
          frame "一级权限", Default {
            n121 = Set Occurrence(w175) -> ()
          }
          frame "二级权限".."超级权限" {
            n122 = flat-sequence {
              tunnel: w176 -> [_]
              frame #0 {
                n123 = global write "CODMn断电保存全局变量.vi" "PORT"("PORT") -> ()
                n124 = global write "CODMn断电保存全局变量.vi" "IP"("IP") -> ()
                n125 = global write "CODMn断电保存全局变量.vi" "流程路径"("流程路径") -> ()
                n126 = global read "CODMn断电保存全局变量.vi" "CODMn关键参数"() -> (w184:T10)
                n127 = global read "CODMn断电保存全局变量.vi" "质控参数设置"() -> (w191:T13)
                n128 = local read "通信方式选择"() -> (w187:enum16{"串口", "TCP"})
                n129 = local read "消解时长"() -> (w186:dbl)
                n130 = global write "CODMn断电保存全局变量.vi" "VISA Resource"("请选择串口:") -> ()
                n131 = Bundle By Name(cluster=w184, "消解时长"=w186) -> (w183:T10)
                n132 = global write "CODMn断电保存全局变量.vi" "MB通信方式选择"(w187) -> ()
                n133 = global write "CODMn断电保存全局变量.vi" "标样核查自动补测"("标样核查自动补测") -> ()
                n134 = global write "CODMn断电保存全局变量.vi" "跨度核查自动补测"("跨度核查自动补测") -> ()
                n135 = global write "CODMn断电保存全局变量.vi" "零点核查自动补测"("零点核查自动补测") -> ()
                n136 = global write "CODMn断电保存全局变量.vi" "CODMn关键参数"(w183) -> ()
                n137 = Bundle By Name(cluster=w191, "跨度值"="跨度值", "零点标准液浓度"="零点核查标液浓度", "跨度标准液浓度"="跨度核查标液浓度", "标准液标准浓度"="标样核查标液浓度", "零点标准液偏差"="零点核查标液偏差", "跨度标准液偏差"="跨度核查标液偏差", "标准液标准偏差"="标样核查标液偏差") -> (w185:T13)
                n138 = global write "CODMn断电保存全局变量.vi" "质控参数设置"(w185) -> ()
              }
              frame #1 {
                n139 = call "配置文件保存.vi"() -> ()  [unwired: 12 in]
              }
            }
          }
        }
      }
      event "自动测试量程配置": Value Change {
        n140 = event-data() -> ()  [unwired: 1 in, 6 out]
        n141 = global read "VARCODMn全局变量.vi" "权限等级"() -> (w198:enum16{"一级权限", "二级权限", "三级权限", "超级权限"})
        n142 = case shown="\"二级权限\"..\"超级权限\"" w198 {
          tunnel: w197 -> [w199 _]
          frame "一级权限", Default {
            n143 = Set Occurrence(w199) -> ()
          }
          frame "二级权限".."超级权限" {
            n144 = flat-sequence {
              frame #0 {
                n145 = global read "VARCODMn全局变量.vi" "MB session in"() -> (w200:refnum<class "MB_Master.lvclass">)
                n146 = call "写入量程参数.vi"("自动测试量程配置"="自动测试量程配置", "MB session in"=w200) -> ()  [unwired: 8 in, 2 out]
                n147 = global write "CODMn断电保存全局变量.vi" "自动测试量程配置"("自动测试量程配置") -> ()
              }
              frame #1 {
                n148 = call "配置文件保存.vi"() -> ()  [unwired: 12 in]
              }
            }
          }
        }
      }
      event "通讯连接": Value Change {
        n149 = event-data() -> ("NewVal"=w202:bool)  [unwired: 1 in, 5 out]
        n150 = Flush Queue(queue=w203) -> (queue out=w204:refnum<queue>)  [unwired: 1 in, 2 out]
        n151 = case shown="真" w202 {
          tunnel: w204 -> [w205 w207]
          frame False {
            n152 = Enqueue Element(queue=w205, element=cluster{"命令":string, "data":variant} {"命令"="停用模块", "data"=variant} ("元素")) -> ()  [unwired: 2 in, 3 out]
          }
          frame True {
            n153 = Enqueue Element(queue=w207, element=cluster{"命令":string, "data":variant} {"命令"="启用模块", "data"=variant} ("元素")) -> ()  [unwired: 2 in, 3 out]
          }
        }
      }
    }
  }
  n154 = while {
    tunnel: w1 -> [w215]
    stop <- FALSE stop-if-true
    n155 = global read "CODMn断电保存全局变量.vi" "PORT"() -> (w229:string)
    n156 = global read "CODMn断电保存全局变量.vi" "IP"() -> (w228:string)
    n157 = Wait (ms)(milliseconds to wait=u32 1000 ("等待时间（毫秒）")) -> ()  [unwired: 1 out]
    n158 = global read "CODMn断电保存全局变量.vi" "流程路径"() -> (w227:path)
    n159 = local write "IP"(w228) -> ()
    n160 = local write "PORT"(w229) -> ()
    n161 = global read "CODMn断电保存全局变量.vi" "零点核查自动补测"() -> (w210:bool)
    n162 = global read "CODMn断电保存全局变量.vi" "跨度核查自动补测"() -> (w209:bool)
    n163 = global read "CODMn断电保存全局变量.vi" "标样核查自动补测"() -> (w214:bool)
    n164 = global read "CODMn断电保存全局变量.vi" "MB通信方式选择"() -> (w226:enum16{"串口", "TCP"})
    n165 = global read "CODMn断电保存全局变量.vi" "VISA Resource"() -> (w230:refnum<visa-resource-name>)
    n166 = local write "流程路径"(w227) -> ()
    n167 = global read "CODMn断电保存全局变量.vi" "质控参数设置"() -> (w221:T13)
    n168 = global read "VARCODMn全局变量.vi" "页面"() -> (w220:enum16{"主页", "参数页", "校准页"})
    n169 = local write "零点核查自动补测"(w210) -> ()
    n170 = local write "跨度核查自动补测"(w209) -> ()
    n171 = local write "标样核查自动补测"(w214) -> ()
    n172 = local write "请选择串口:"(w230) -> ()
    n173 = Unbundle By Name(w221) -> ("跨度值"=w222:dbl, "零点标准液浓度"=w223:dbl, "跨度标准液浓度"=w224:dbl, "标准液标准浓度"=w225:dbl, "零点标准液偏差"=w213:dbl, "跨度标准液偏差"=w212:dbl, "标准液标准偏差"=w211:dbl)
    n174 = local write "通信方式选择"(w226) -> ()
    n175 = Equal?(x=w220, y=enum16{"主页", "参数页", "校准页"}."参数页") -> (x = y?=w218:bool)
    n176 = local write "跨度值"(w222) -> ()
    n177 = local write "零点核查标液浓度"(w223) -> ()
    n178 = local write "跨度核查标液浓度"(w224) -> ()
    n179 = local write "标样核查标液浓度"(w225) -> ()
    n180 = local write "零点核查标液偏差"(w213) -> ()
    n181 = local write "跨度核查标液偏差"(w212) -> ()
    n182 = local write "标样核查标液偏差"(w211) -> ()
    n183 = call <vilib>:"Boolean Crossing PtByPt.vi"("direction"=enum16{"either", "false-true", "true-false"}."false-true", "input"=w218) -> ("crossing"=w216:bool)  [unwired: 1 in]
    n184 = case shown="真" w216 {
      tunnel: w215 -> [_ w233]
      frame False {
      }
      frame True {
        n185 = Set Occurrence(w233) -> ()
      }
    }
  }
  n186 = while {
    tunnel: w3 -> [w245]
    tunnel: w4 -> [w244]
    tunnel: w5 -> [w243]
    tunnel: w1 -> [w242]
    stop <- FALSE stop-if-true
    n187 = Wait on Occurrence(2:w242) -> (0:w236:bool)  [unwired: 2 in]
    n188 = flat-sequence {
      tunnel: w245 -> [w252]
      tunnel: w244 -> [w251]
      tunnel: w243 -> [w250]
      tunnel: [w249] -> w239
      tunnel: [w248] -> w238
      tunnel: [w247] -> w237
      tunnel: w236 -> [_]
      frame #0 {
        n189 = property class="Enum (严格)"(reference=w250) -> ("Value"=w247:T3)  [unwired: 1 in, 2 out]
        n190 = property class="Enum (严格)"(reference=w251) -> ("Value"=w248:enum16{"低量程", "高量程"})  [unwired: 1 in, 2 out]
        n191 = property class="Ring (严格)"(reference=w252) -> ("Value"=w249:u16)  [unwired: 1 in, 2 out]
      }
    }
    n192 = flat-sequence {
      tunnel: [w255] -> w241
      tunnel: [w254] -> w240
      tunnel: w239 -> [w253]
      tunnel: w238 -> [w255]
      tunnel: w237 -> [w254]
      tunnel: [w253] -> w234
      tunnel: w241 -> [w263]
      tunnel: w240 -> [w266]
      tunnel: [w264] -> w235
      tunnel: w234 -> [_]
      tunnel: w235 -> [w293]
      frame #0 {
      }
      frame #1 {
        n193 = case shown="\"低量程\", 默认" w263 {
          tunnel: [enum16{"低量程1", "低量程2", "高量程1", "高量程2"}."低量程1" ("量程") enum16{"低量程1", "低量程2", "高量程1", "高量程2"}."高量程1" ("量程")] -> w262
          tunnel: [enum16{"低量程1", "低量程2", "高量程1", "高量程2"}."低量程2" ("量程") enum16{"低量程1", "低量程2", "高量程1", "高量程2"}."高量程2" ("量程")] -> w261
          frame "低量程", Default {
          }
          frame "高量程" {
          }
        }
        n194 = global read "CODMn断电保存全局变量.vi" "CODMn关键参数"() -> (w271:T10)
        n195 = global read "VARCODMn全局变量.vi" "MB session in"() -> (w273:refnum<class "MB_Master.lvclass">)
        n196 = Unbundle By Name(w271) -> ("消解温度"=→"消解温度":sgl, "消解时长"=→"消解时长":sgl)
        n197 = call "读取量程参数.vi"("引用选择"=enum16{"MB引用", "自建引用"}."MB引用", "MB session in"=w273) -> ("error out"=w269:errorcluster, "自动测试量程配置"=w256:T2, "MB session out"=w268:refnum<class "MB_Master.lvclass">)  [unwired: 7 in]
        n198 = local write "自动测试量程配置"(w256) -> ()
        n199 = global write "CODMn断电保存全局变量.vi" "自动测试量程配置"(w256) -> ()
        n200 = call "读取内置参数.vi"("error in (no error)"=w269, "MB session in"=w268) -> ("error out"=w270:errorcluster, "量程参数读取"=w274:T6)  [unwired: 5 in, 3 out]
        n201 = Unbundle By Name(w274) -> ("测量精度"=→"测量精度":dbl, "检出限"=→"检出限":dbl, "上限"=→"量程上限":dbl, "下限"=→"量程下限":dbl, "阈值（低->高）"=→"阈值（低->高）":dbl, "阈值（高->低）"=→"阈值（高->低）":dbl)
        n202 = call "公式读取.vi"("error in (no error)"=w270, "量程"=w262, "测量模式"=w266, "测量参数"=enum16{"CODMn"}."CODMn") -> ("error out"=w265:errorcluster, "临界滴定数"=w276:dbl, "公式"=w282:cluster{"X^2":dbl, "X":dbl, "b":dbl})  [unwired: 5 in]
        n203 = Unbundle By Name(w282) -> ("X^2"=→"二次多项式系数":dbl, "X"=→"曲线斜率":dbl, "b"=→"曲线截距":dbl)
        n204 = local write "公式切换阈值滴定数(0~9999)"(w276) -> ()
        n205 = call "公式读取.vi"("error in (no error)"=w265, "量程"=w261, "测量模式"=w266, "测量参数"=enum16{"CODMn"}."CODMn") -> ("error out"=w264:errorcluster, "公式"=w260:cluster{"X^2":dbl, "X":dbl, "b":dbl})  [unwired: 5 in, 1 out]
        n206 = Unbundle By Name(w260) -> ("X^2"=→"二次多项式系数 2":dbl, "X"=→"曲线斜率 2":dbl, "b"=→"曲线截距 2":dbl)
      }
      frame #2 {
        n207 = Format Date/Time String() -> (date/time string=→"数据刷新时间":string)  [unwired: 3 in]
        "error out" <- w293
      }
    }
  }
